vi "Set Value.vi"(8 "error in (no error)":errorcluster, 10 "Value":refnum<class>, 11 "PathTreeNode in":refnum<class "PathTreeNode.lvclass">) -> (0 "error out":errorcluster, 3 "PathTreeNode out":refnum<class "PathTreeNode.lvclass">)   [LabVIEW 2020, in "Advanced Structures.lvlib" / "PathTreeNode.lvclass"]
uses:
  PathTreeNode.lvclass
  PathTreeNode.lvclass/PathTreeNode.ctl
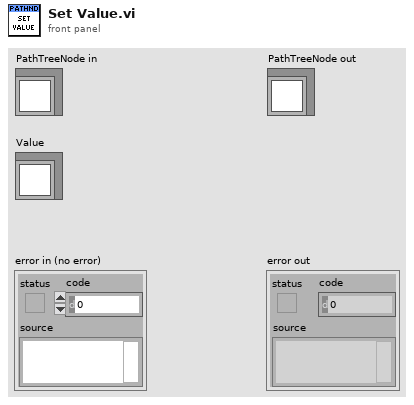
[diagram p1: front panel]
types:
  T1 = typedef "Advanced Structures.lvlib/PathTreeNode.lvclass/Ref Data.ctl" = cluster{"Tree":refnum<class>, "Parent":refnum<class>, "Token":string, "Child Tokens":string[], "Child Nodes":refnum<class>[], "Value":refnum<class>, "Has Value":bool}
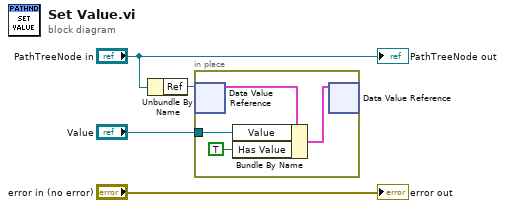
[diagram p0: block diagram]
diagram:
  n1 = Unbundle By Name("PathTreeNode in") -> ("Ref"=w3:refnum<data-value>)
  n2 = in-place {
    in-place-border: "Value" -> [w6]
    n3 = in-place-dvr #1(w3) -> (w8:T1)  [unwired: 1 out]
    n4 = Bundle By Name(cluster=w8, "Value"=w6, "Has Value"=TRUE) -> (w7:T1)
    n5 = in-place-dvr #1(w7) -> ()  [unwired: 2 out]
  }
  "error out" <- "error in (no error)"
  "PathTreeNode out" <- "PathTreeNode in"
